vi "get_or_set_pattern.vi"(7 "action":T1, 8 "error in (no error)":errorcluster, 10 "samples in":dbl[](array[numeric]), 11 "Stimulator090724 in":refnum<class "Stimulator090724Scaffold.lvclass">) -> (0 "error out":errorcluster, 2 "samples out":dbl[](array[numeric]), 3 "Stimulator090724 out":refnum<class "Stimulator090724Scaffold.lvclass">)   [LabVIEW 2010, in "Stimulator090724Scaffold.lvclass"]
uses:
  Stimulator090724Scaffold.lvclass
  common/enumerations/functional_global_action_enum.ctl
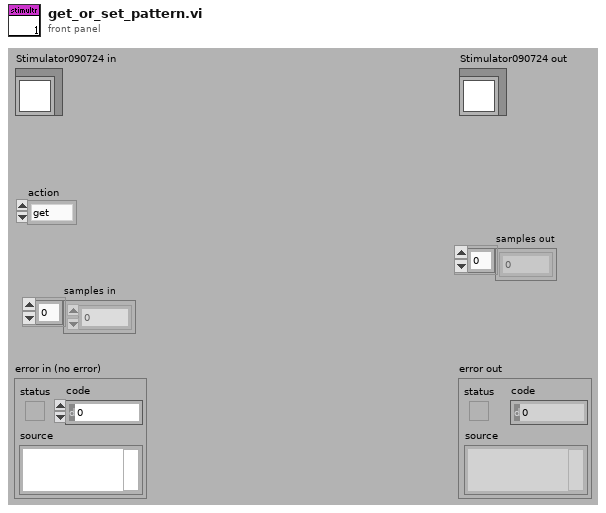
[diagram p1: front panel]
types:
  T1 = typedef "functional_global_action_enum.ctl" = enum16{"get", "set", "reset"}
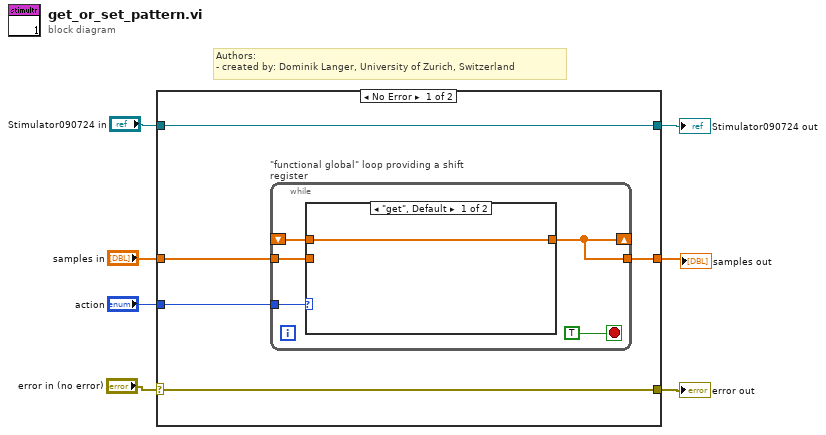
[diagram p0: block diagram]
diagram:
  # "Authors: \n- created by: Dominik Langer, University of Zurich, Switzerland"
  n1 = case shown="No Error" "error in (no error)" {
    selector: "error in (no error)" -> [w11 w21]
    tunnel: [w11 w21] -> w6
    tunnel: [w12 w20] -> w4
    tunnel: "Stimulator090724 in" -> [w12 w20]
    tunnel: "action" -> [w10 _]
    tunnel: "samples in" -> [w9 _]
    tunnel: [w8 _] -> w1
    frame No Error {
      n2 = while "\"functional global\" loop providing a shift register" {
        shift-right: [w13] -> _
        shift-left: _ -> [w14]
        tunnel: w10 -> [w16]
        tunnel: w9 -> [w15]
        tunnel: [w13] -> w8
        stop <- TRUE stop-if-true
        n3 = case shown="\"get\", Default" w16 {
          tunnel: w15 -> [_ w19]
          tunnel: [w18 w19] -> w13
          tunnel: w14 -> [w18 _]
          frame "get", Default {
          }
          frame "set" {
          }
        }
      }
    }
    frame Error {
    }
  }
  "error out" <- w6
  "Stimulator090724 out" <- w4
  "samples out" <- w1
